vi "generate tomo compatible file name.vi"(7 "Numeric":i32, 8 "error in (no error)":errorcluster, 11 "Thorcam in":refnum<class "Thorcam.lvclass">) -> (0 "error out":errorcluster, 1 "String":string, 3 "Thorcam out":refnum<class "Thorcam.lvclass">)   [LabVIEW 2012, in "Thorcam.lvclass"]
uses:
  Thorcam.lvclass
  Thorcam.lvclass/Thorcam.ctl
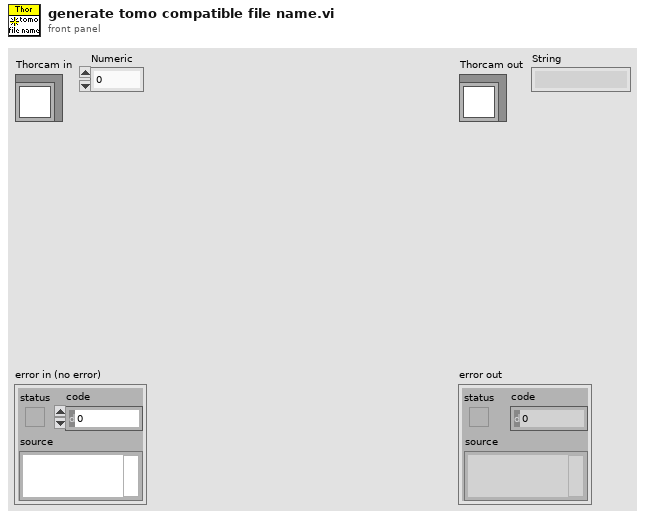
[diagram p1: front panel]
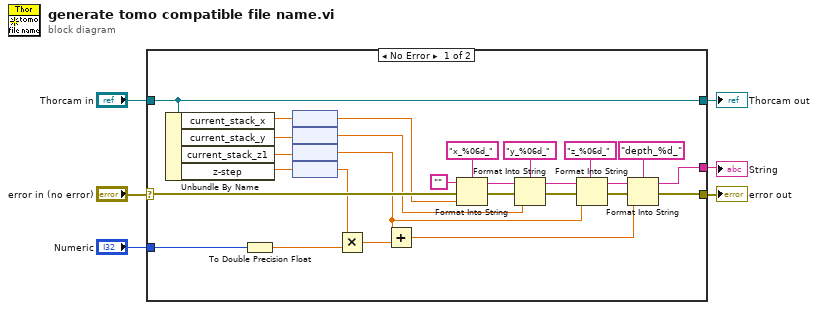
[diagram p0: block diagram]
diagram:
  n1 = case shown="No Error" "error in (no error)" {
    selector: "error in (no error)" -> [w22 w35]
    tunnel: [w21 w35] -> w5
    tunnel: [w33 w34] -> w3
    tunnel: "Thorcam in" -> [w33 w34]
    tunnel: [w13 _] -> w2
    tunnel: "Numeric" -> [w12 _]
    frame No Error {
      n2 = Unbundle By Name(w33) -> ("current_stack_x"=w19:dbl[unit], "current_stack_y"=w17:dbl[unit], "current_stack_z1"=w16:dbl[unit], "z-step"=w15:dbl[unit])
      n3 = To Double Precision Float(number=w12) -> (double precision float=w11:dbl)
      n4 = node(w19) -> (w18:dbl)
      n5 = node(w17) -> (w14:dbl)
      n6 = node(w16) -> (w8:dbl)
      n7 = node(w15) -> (w10:dbl)
      n8 = Multiply(x=w10, y=w11) -> (x*y=w9:dbl)
      n9 = Add(x=w8, y=w9) -> (x+y=w7:dbl)
      n10 = Format Into String(format string="x_%06d_", initial string="", error in=w22, w18) -> (resulting string=w27:string, error out=w24:errorcluster)
      n11 = Format Into String(format string="y_%06d_", initial string=w27, error in=w24, w14) -> (resulting string=w28:string, error out=w25:errorcluster)
      n12 = Format Into String(format string="z_%06d_", initial string=w28, error in=w25, w8) -> (resulting string=w29:string, error out=w26:errorcluster)
      n13 = Format Into String(format string="depth_%d_", initial string=w29, error in=w26, w7) -> (resulting string=w13:string, error out=w21:errorcluster)
    }
    frame Error {
    }
  }
  "error out" <- w5
  "Thorcam out" <- w3
  "String" <- w2
